vi "DIO board parameters global.vi"() -> ()   [LabVIEW 2017]
panel:
  in  "# of lines":u16=32
  in  "Data to the board":u32[][](array[numeric])
  in  "Mask":u16[](array[numeric])=[65535] format="%.0x"
  in  "# of ports":u16=4
  in  "Initial data":u16[][](array[numeric])=[[0, 6, 1]] format="%.0b"
  in  "Clock Frequency":dbl=1000000.0 format="%.2f"
  in  "Base I/O":u16=384 format="%.0x"
  in  "Board":u16
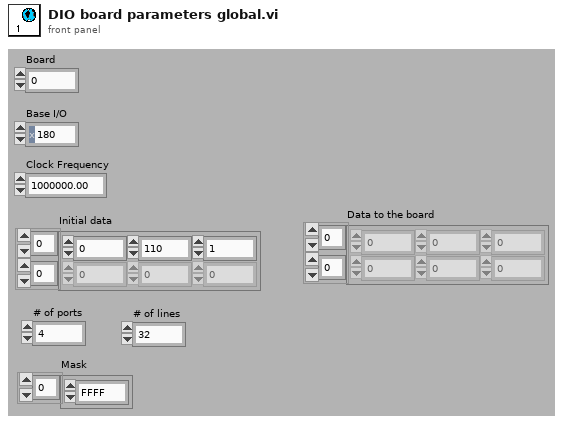
[diagram p1: front panel]
diagram:
